vi "Set Configuration Option.vi"(8 "Line Config 3":bool[](array[boolean]), 9 "Line Config 2":bool[](array[boolean]), 10 "Line Config 1":bool[](array[boolean]), 11 "Line Config 0":bool[](array[boolean])) -> (3 "Configuration Options":T1(ring))   [LabVIEW 2014, in "SLSC configuration System Explorer.lvlib"]
uses:
  SLSC configuration System Explorer.lvlib
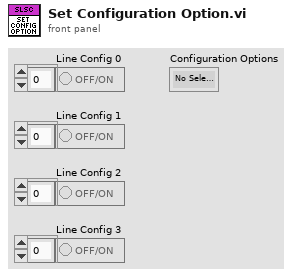
[diagram p1: front panel]
types:
  T1 = enum32{"No Selection", "All Inputs", "All Outputs"}
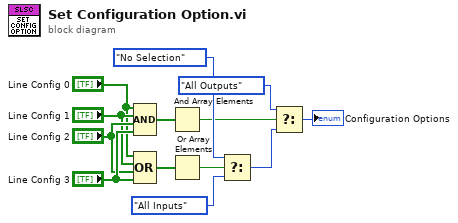
[diagram p0: block diagram]
diagram:
  n1 = Compound Arithmetic op=AND("Line Config 0", "Line Config 1", "Line Config 2", "Line Config 3") -> (w4:bool[])
  n2 = Compound Arithmetic op=OR("Line Config 0", "Line Config 1", "Line Config 2", "Line Config 3") -> (w9:bool[])
  n3 = And Array Elements(Boolean array=w4) -> (logical AND=w1:bool)
  n4 = Or Array Elements(Boolean array=w9) -> (logical OR=w10:bool)
  n5 = Select(t=T1."No Selection" ("Configuration Options"), s=w10, f=T1."All Inputs" ("Configuration Options")) -> (s? t:f=w13:T1)
  n6 = Select(t=T1."All Outputs" ("Configuration Options"), s=w1, f=w13) -> (s? t:f=→"Configuration Options":T1)
